vi "Close handle.vi"(1 "Device Handle":u64) -> (0 "Error":errorcluster)   [LabVIEW 2018]
uses:
  Coherent global.vi
panel:
  # "PN 06/11/2014\n      08/04/2019"
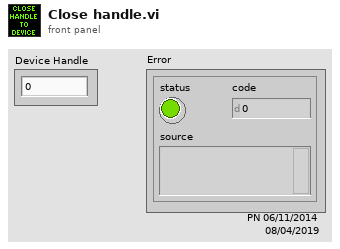
[diagram p1: front panel]
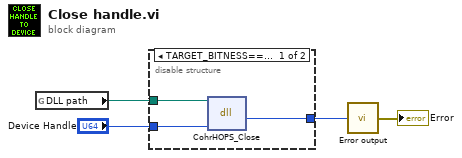
[diagram p0: block diagram]
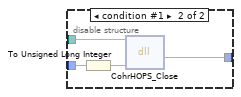
[diagram p2: hidden frame]
diagram:
  n1 = global read "Coherent global.vi" "DLL path"() -> (w1:path)
  n2 = disable-structure shown="TARGET_BITNESS==64" {
    disable-tunnel: "Device Handle" -> [w7 w11]
    disable-tunnel: [w6 w9] -> w3
    disable-tunnel: w1 -> [w5 w10]
    frame condition #0 (active) {
      n3 = dll-call lib="?" fn="CohrHOPS_Close"(path in=w5, "handle"=w7) -> ("return type"=w6:i32)  [unwired: 3 in, 2 out]
    }
    frame condition #1 {
      n4 = To Unsigned Long Integer(number=w11) -> (unsigned 32bit integer=w8:u32)
      n5 = dll-call lib="?" fn="CohrHOPS_Close"(path in=w10, "handle"=w8) -> ("return type"=w9:i32)  [unwired: 3 in, 2 out]
    }
  }
  n6 = call "Error output.vi"("I32 err code"=w3) -> ("Error Out"=→"Error":errorcluster)
